vi "Pct-Encode String.vi"(4 "String":string) -> (7 "Pct-Encoded String":string)   [LabVIEW 2020, in "URI.lvlib"]
uses:
  URI.lvlib
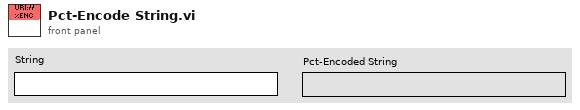
[diagram p1: front panel]
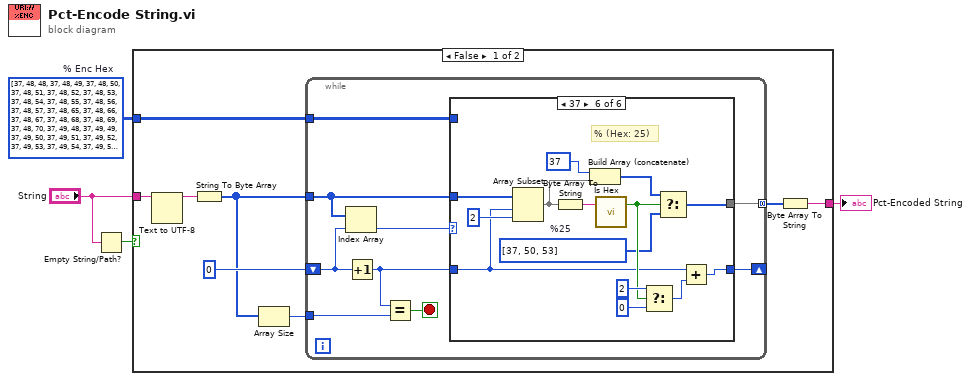
[diagram p0: block diagram]
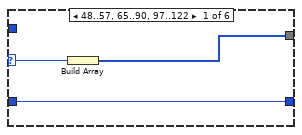
[diagram p2: hidden frame]
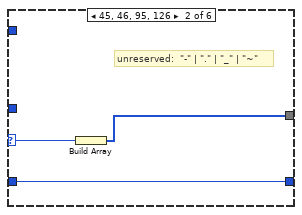
[diagram p3: hidden frame]
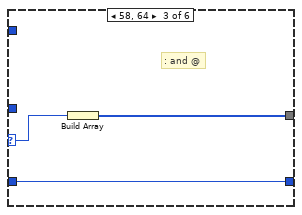
[diagram p4: hidden frame]
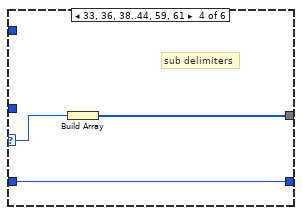
[diagram p5: hidden frame]
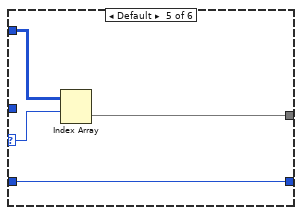
[diagram p6: hidden frame]
diagram:
  w1 = u8[][] [[37, 48, 48], [37, 48, 49], [37, 48, 50], [37, 48, 51], [37, 48, 52], [37, 48, 53], [37, 48, 54], [37, 48, 55], [37, 48, 56], [37, 48, 57], [37, 48, 65], [37, 48, 66], [37, 48, 67], [37, 48, 68], [37, 48, 69], [37, 48, 70], [37, 49, 48], [37, 49, 49], [37, 49, 50], [37, 49, 51], [37, 49, 52], [37, 49, 53], [37, 49, 54], [37, 49, 55], [37, 49, 56], [37, 49, 57], [37, 49, 65], [37, 49, 66], [37, 49, 67], [37, 49, 68], [37, 49, 69], [37, 49, 70], [37, 50, 48], [37, 50, 49], [37, 50, 50], [37, 50, 51], [37, 50, 52], [37, 50, 53], [37, 50, 54], [37, 50, 55], [37, 50, 56], [37, 50, 57], [37, 50, 65], [37, 50, 66], [37, 50, 67], [37, 50, 68], [37, 50, 69], [37, 50, 70], [37, 51, 48], [37, 51, 49], [37, 51, 50], [37, 51, 51], [37, 51, 52], [37, 51, 53], [37, 51, 54], [37, 51, 55], [37, 51, 56], [37, 51, 57], [37, 51, 65], [37, 51, 66], [37, 51, 67], [37, 51, 68], [37, 51, 69], [37, 51, 70], [37, 52, 48], [37, 52, 49], [37, 52, 50], [37, 52, 51], [37, 52, 52], [37, 52, 53], [37, 52, 54], [37, 52, 55], [37, 52, 56], [37, 52, 57], [37, 52, 65], [37, 52, 66], [37, 52, 67], [37, 52, 68], [37, 52, 69], [37, 52, 70], [37, 53, 48], [37, 53, 49], [37, 53, 50], [37, 53, 51], [37, 53, 52], [37, 53, 53], [37, 53, 54], [37, 53, 55], [37, 53, 56], [37, 53, 57], [37, 53, 65], [37, 53, 66], [37, 53, 67], [37, 53, 68], [37, 53, 69], [37, 53, 70], [37, 54, 48], [37, 54, 49], [37, 54, 50], [37, 54, 51], [37, 54, 52], [37, 54, 53], [37, 54, 54], [37, 54, 55], [37, 54, 56], [37, 54, 57], [37, 54, 65], [37, 54, 66], [37, 54, 67], [37, 54, 68], [37, 54, 69], [37, 54, 70], [37, 55, 48], [37, 55, 49], [37, 55, 50], [37, 55, 51], [37, 55, 52], [37, 55, 53], [37, 55, 54], [37, 55, 55], [37, 55, 56], [37, 55, 57], [37, 55, 65], [37, 55, 66], [37, 55, 67], [37, 55, 68], [37, 55, 69], [37, 55, 70], [37, 56, 48], [37, 56, 49], [37, 56, 50], [37, 56, 51], [37, 56, 52], [37, 56, 53], [37, 56, 54], [37, 56, 55], [37, 56, 56], [37, 56, 57], [37, 56, 65], [37, 56, 66], [37, 56, 67], [37, 56, 68], [37, 56, 69], [37, 56, 70], [37, 57, 48], [37, 57, 49], [37, 57, 50], [37, 57, 51], [37, 57, 52], [37, 57, 53], [37, 57, 54], [37, 57, 55], [37, 57, 56], [37, 57, 57], [37, 57, 65], [37, 57, 66], [37, 57, 67], [37, 57, 68], [37, 57, 69], [37, 57, 70], [37, 65, 48], [37, 65, 49], [37, 65, 50], [37, 65, 51], [37, 65, 52], [37, 65, 53], [37, 65, 54], [37, 65, 55], [37, 65, 56], [37, 65, 57], [37, 65, 65], [37, 65, 66], [37, 65, 67], [37, 65, 68], [37, 65, 69], [37, 65, 70], [37, 66, 48], [37, 66, 49], [37, 66, 50], [37, 66, 51], [37, 66, 52], [37, 66, 53], [37, 66, 54], [37, 66, 55], [37, 66, 56], [37, 66, 57], [37, 66, 65], [37, 66, 66], [37, 66, 67], [37, 66, 68], [37, 66, 69], [37, 66, 70], [37, 67, 48], [37, 67, 49], [37, 67, 50], [37, 67, 51], [37, 67, 52], [37, 67, 53], [37, 67, 54], [37, 67, 55], [37, 67, 56], [37, 67, 57], [37, 67, 65], [37, 67, 66], [37, 67, 67], [37, 67, 68], [37, 67, 69], [37, 67, 70], [37, 68, 48], [37, 68, 49], [37, 68, 50], [37, 68, 51], [37, 68, 52], [37, 68, 53], [37, 68, 54], [37, 68, 55], [37, 68, 56], [37, 68, 57], [37, 68, 65], [37, 68, 66], [37, 68, 67], [37, 68, 68], [37, 68, 69], [37, 68, 70], [37, 69, 48], [37, 69, 49], [37, 69, 50], [37, 69, 51], [37, 69, 52], [37, 69, 53], [37, 69, 54], [37, 69, 55], [37, 69, 56], [37, 69, 57], [37, 69, 65], [37, 69, 66], [37, 69, 67], [37, 69, 68], [37, 69, 69], [37, 69, 70], [37, 70, 48], [37, 70, 49], [37, 70, 50], [37, 70, 51], [37, 70, 52], [37, 70, 53], [37, 70, 54], [37, 70, 55], [37, 70, 56], [37, 70, 57], [37, 70, 65], [37, 70, 66], [37, 70, 67], [37, 70, 68], [37, 70, 69], [37, 70, 70]]  # % Enc Hex
  n1 = Empty String/Path?(string/path="String") -> (empty?=w3:bool)
  n2 = case shown="False" w3 {
    tunnel: "String" -> [w12 _]
    tunnel: [w9 _] -> w4
    tunnel: w1 -> [w7 _]
    frame False {
      n3 = Text to UTF-8(11:w12) -> (3:w11:string)  [unwired: 2 in, 1 out]
      n4 = String To Byte Array(string=w11) -> (unsigned byte array=w6:u8[])
      n5 = Array Size(array=w6) -> (size(s)=w5:i32)
      n6 = while {
        tunnel: [w21] -> w10 mode=concatenating
        tunnel: w6 -> [w17]
        shift-right: [w18] -> _
        shift-left: 0 -> [w19]
        tunnel: w7 -> [w16]
        tunnel: w5 -> [w14]
        stop <- w13 stop-if-true
        n7 = Index Array(array=w17, index=w19) -> (element=w20:u8)
        n8 = Increment(x=w19) -> (x+1=w15:i32)
        n9 = Equal?(x=w15, y=w14) -> (x = y?=w13:bool)
        n10 = case shown="37" w20 {
          selector: w20 -> [w24 w27 w30 w33 w35 _]
          tunnel: [w22 w26 w29 w32 w34 w51] -> w21
          tunnel: w15 -> [w23 w25 w28 w31 w37 w41]
          tunnel: [w23 w25 w28 w31 w37 w45] -> w18
          tunnel: w17 -> [_ _ _ _ _ w49]
          tunnel: w16 -> [_ _ _ _ w36 _]
          frame 48..57, 65..90, 97..122 {
            n11 = Build Array(w24) -> (w22:u8[])
          }
          frame 45, 46, 95, 126 {
            # "unreserved:  \"-\" | \".\" | \"_\" | \"~\""
            n12 = Build Array(w27) -> (w26:u8[])
          }
          frame 58, 64 {
            # ": and @"
            n13 = Build Array(w30) -> (w29:u8[])
          }
          frame 33, 36, 38..44, 59, 61 {
            # "sub delimiters"
            n14 = Build Array(w33) -> (w32:u8[])
          }
          frame Default {
            n15 = Index Array(array=w36, index (row)=w35) -> (element=w34:u8[])  [unwired: 1 in]
          }
          frame 37 {
            w42 = u8[] [37, 50, 53]  # %25
            # "% (Hex: 25)"
            n16 = Array Subset(array=w49, index=w41, length=2) -> (w39:u8[])
            n17 = Byte Array To String(unsigned byte array=w39) -> (string=w50:string)
            n18 = Build Array (concatenate)(u8 37 ("%"), w39) -> (w38:u8[])
            n19 = call "Is Hex.vi"("String"=w50) -> ("Hex"=w44:bool)  [unwired: 6 in]
            n20 = Select(t=2, s=w44, f=0) -> (s? t:f=w43:i32)
            n21 = Select(t=w38, s=w44, f=w42) -> (s? t:f=w51:u8[])
            n22 = Add(x=w41, y=w43) -> (x+y=w45:i32)
          }
        }
      }
      n23 = Byte Array To String(unsigned byte array=w10) -> (string=w9:string)
    }
    frame True {
    }
  }
  "Pct-Encoded String" <- w4
